vi "initqueuename.vi"(0 "object in":refnum<class "interface.lvclass">, 5 "error in (no error)":errorcluster) -> (14 "object out":refnum<class "interface.lvclass">, 19 "error out":errorcluster)   [LabVIEW 2016, in "interface.lvclass"]
uses:
  interface.lvclass
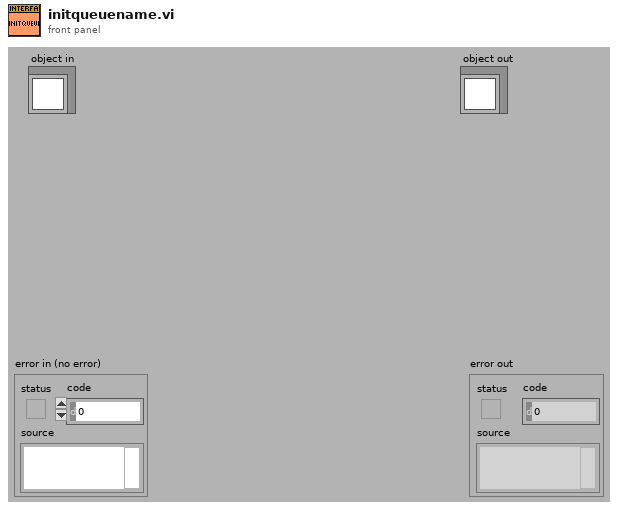
[diagram p1: front panel]
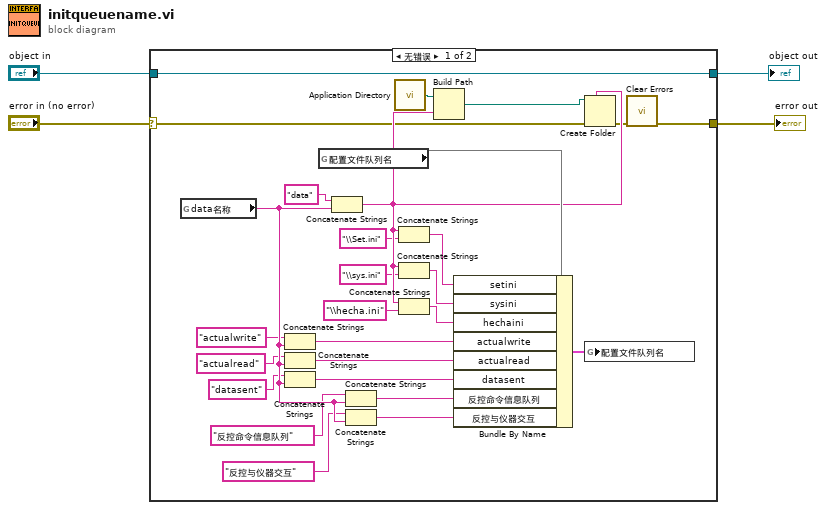
[diagram p0: block diagram]
diagram:
  n1 = case shown="无错误" "error in (no error)" {
    selector: "error in (no error)" -> [w6 w33]
    tunnel: [w5 w33] -> w3
    tunnel: [w31 w32] -> w1
    tunnel: "object in" -> [w31 w32]
    frame No Error {
      n2 = global read "断电保存全局.vi" "data名称"() -> (w28:string)
      n3 = Concatenate Strings("actualwrite" ("名称（未命名）"), w28) -> (w19:string)
      n4 = Concatenate Strings("actualread" ("名称（未命名）"), w28) -> (w21:string)
      n5 = Concatenate Strings("datasent" ("名称（未命名）"), w28) -> (w23:string)
      n6 = global read "断电保存全局.vi" "配置文件队列名"() -> (w29)
      n7 = Concatenate Strings("data" ("对话框窗口（创建文件夹）"), w28) -> (w14:string)
      n8 = Concatenate Strings("反控命令信息队列" ("名称（未命名）"), w28) -> (w27:string)
      n9 = Concatenate Strings("反控与仪器交互" ("名称（未命名）"), w28) -> (w26:string)
      n10 = call <vilib>:"Application Directory.vi"() -> ("Application Directory"=w8:path)
      n11 = Concatenate Strings(w14, "\\Set.ini" ("名称或相对路径")) -> (w12:string)
      n12 = Concatenate Strings(w14, "\\sys.ini" ("名称或相对路径")) -> (w15:string)
      n13 = Concatenate Strings(w14, "\\hecha.ini" ("名称或相对路径")) -> (w16:string)
      n14 = Build Path(base path=w8, name or relative path=w14) -> (appended path=w9:path)
      n15 = Bundle By Name(cluster=w29, "setini"=w12, "sysini"=w15, "hechaini"=w16, "actualwrite"=w19, "actualread"=w21, "datasent"=w23, "反控命令信息队列"=w27, "反控与仪器交互"=w26) -> (w30:cluster{})
      n16 = Create Folder(prompt (Create Folder)=w14, path (use dialog)=w9, error in=w6) -> (error out=w10:errorcluster)  [unwired: 2 out]
      n17 = global write "断电保存全局.vi" "配置文件队列名"(w30) -> ()
      n18 = call <vilib>:"Clear Errors.vi"("error in (no error)"=w10) -> ("error out"=w5:errorcluster)  [unwired: 5 in, 1 out]
    }
    frame Error {
    }
  }
  "error out" <- w3
  "object out" <- w1
